vi "均衡参数输入.vi"(1 "均衡参数":T2 {"充电结束电压(100%)" min=0 max=5 format="%#.4f"; "充电结束电压(99%)" min=0 max=5 format="%#.4f"; "充电结束电压(98%)" min=0 max=5 format="%#.4f"; "充电结束电压(97%)" min=0 max=5 format="%#.4f"; "充电结束电压(96%)" min=0 max=5 format="%#.4f"; "充电结束电压(95%)" min=0 max=5 format="%#.4f"; "均衡计算-电压极差阀值" min=0 max=5 format="%#.4f"; "均衡停止-最低电压阀值" min=0 max=5 format="%#.4f"; "均衡计算-最低电压阀值" min=0 max=5 format="%#.4f"; "均衡计算-电压低阀值2级" min=0 max=5 format="%#.4f"; "充电结束电压(94%)" min=0 max=5 format="%#.4f"; "充电结束电压(93%)" min=0 max=5 format="%#.4f"; "均衡计算-电压低阀值1级" min=0 max=5 format="%#.4f"; "均衡计算-电压高阀值1级" min=0 max=5 format="%#.4f"; "均衡计算-电压高阀值2级" min=0 max=5 format="%#.4f"; "充电结束电压(92%)" min=0 max=5 format="%#.4f"; "充电结束电压(91%)" min=0 max=5 format="%#.4f"; "充电结束电压(90%)" min=0 max=5 format="%#.4f"}) -> (0 "均衡参数 2":T1 {"充电结束电压(100%)" min=0 max=5 format="%#.4f"; "充电结束电压(99%)" min=0 max=5 format="%#.4f"; "充电结束电压(98%)" min=0 max=5 format="%#.4f"; "充电结束电压(97%)" min=0 max=5 format="%#.4f"; "充电结束电压(96%)" min=0 max=5 format="%#.4f"; "充电结束电压(95%)" min=0 max=5 format="%#.4f"; "均衡计算-电压极差阀值" min=0 max=5 format="%#.4f"; "均衡停止-最低电压阀值" min=0 max=5 format="%#.4f"; "均衡计算-最低电压阀值" min=0 max=5 format="%#.4f"; "均衡计算-电压低阀值2级" min=0 max=5 format="%#.4f"; "充电结束电压(94%)" min=0 max=5 format="%#.4f"; "充电结束电压(93%)" min=0 max=5 format="%#.4f"; "均衡计算-电压低阀值1级" min=0 max=5 format="%#.4f"; "均衡计算-电压高阀值1级" min=0 max=5 format="%#.4f"; "均衡计算-电压高阀值2级" min=0 max=5 format="%#.4f"; "充电结束电压(92%)" min=0 max=5 format="%#.4f"; "充电结束电压(91%)" min=0 max=5 format="%#.4f"; "充电结束电压(90%)" min=0 max=5 format="%#.4f"})   [LabVIEW 2013]
panel:
  in  "全部输入..":bool
  in  "停止":bool
  in  "确定":bool
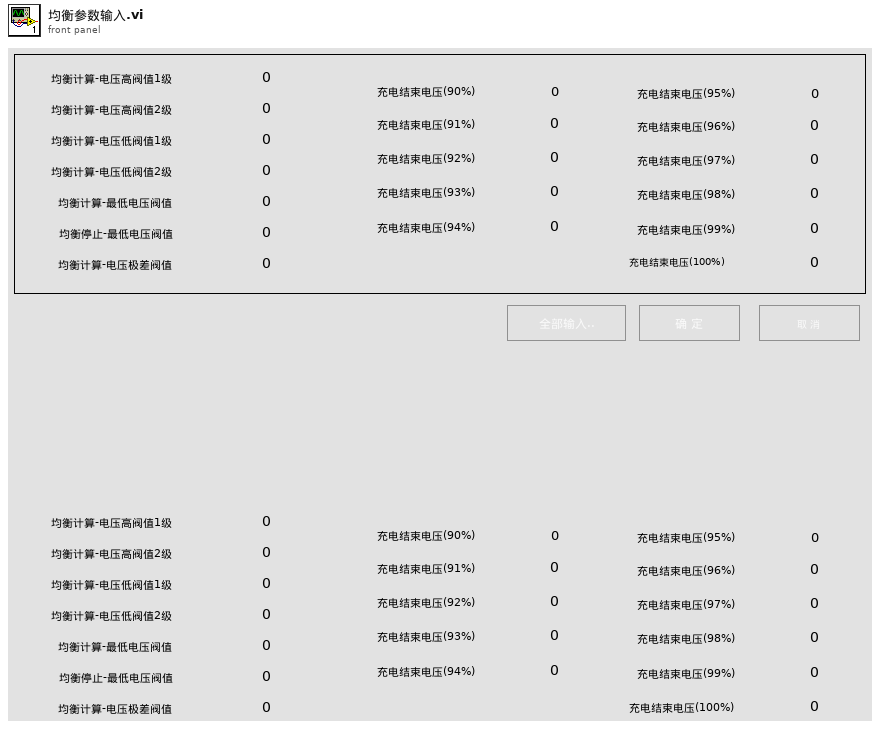
[diagram p1: front panel]
types:
  T1 = cluster{"充电结束电压(90%)":sgl, "充电结束电压(91%)":sgl, "充电结束电压(92%)":sgl, "充电结束电压(93%)":sgl, "充电结束电压(94%)":sgl, "均衡计算-电压高阀值1级":sgl, "均衡计算-电压高阀值2级":sgl, "均衡计算-电压低阀值1级":sgl, "均衡计算-电压低阀值2级":sgl, "均衡计算-最低电压阀值":sgl, "均衡停止-最低电压阀值":sgl, "均衡计算-电压极差阀值":sgl, "充电结束电压(95%)":sgl, "充电结束电压(96%)":sgl, "充电结束电压(97%)":sgl, "充电结束电压(98%)":sgl, "充电结束电压(99%)":sgl, "充电结束电压(100%)":sgl}
  T2 = cluster{"均衡计算-电压高阀值1级":sgl, "均衡计算-电压高阀值2级":sgl, "均衡计算-电压低阀值1级":sgl, "均衡计算-电压低阀值2级":sgl, "均衡计算-最低电压阀值":sgl, "均衡停止-最低电压阀值":sgl, "均衡计算-电压极差阀值":sgl, "充电结束电压(90%)":sgl, "充电结束电压(91%)":sgl, "充电结束电压(92%)":sgl, "充电结束电压(93%)":sgl, "充电结束电压(94%)":sgl, "充电结束电压(95%)":sgl, "充电结束电压(96%)":sgl, "充电结束电压(97%)":sgl, "充电结束电压(98%)":sgl, "充电结束电压(99%)":sgl, "充电结束电压(100%)":sgl}
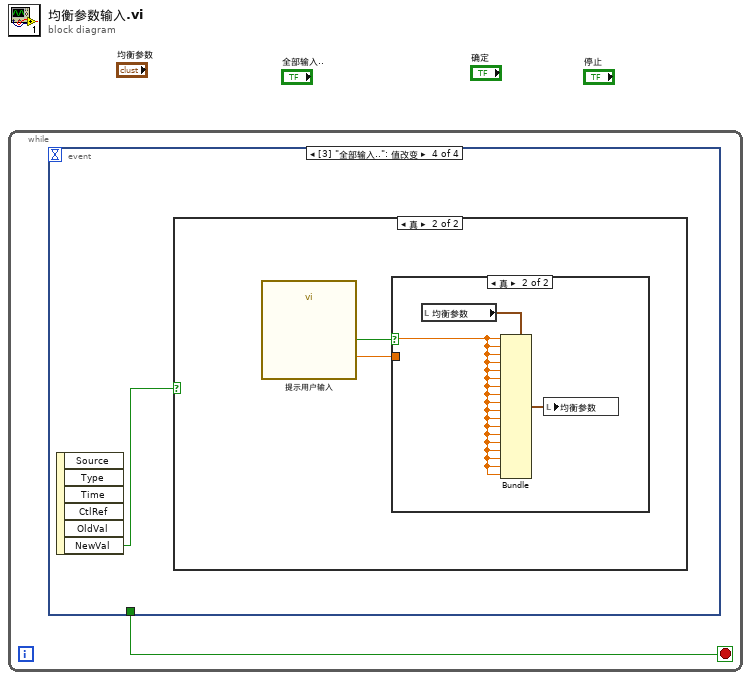
[diagram p0: block diagram]
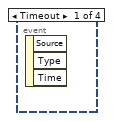
[diagram p2: hidden frame]
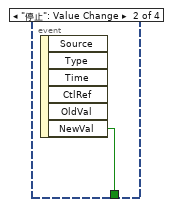
[diagram p3: hidden frame]
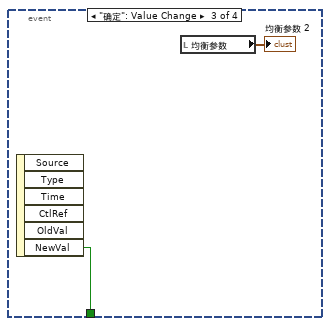
[diagram p4: hidden frame]
diagram:
  n1 = while {
    stop <- w1 stop-if-true
    n2 = event shown="[3] \"全部输入..\": 值改变" {
      selector: _ -> [_ _ _ _]
      dyn-events: _ -> [_ _ _ _]
      timeout: _ -> [_ _ _ _]
      tunnel: [_ w2 w4 _] -> w1
      event Timeout {
        n3 = event-data() -> ()  [unwired: 1 in, 3 out]
      }
      event "停止": Value Change {
        n4 = event-data() -> ("NewVal"=w2:bool)  [unwired: 1 in, 5 out]
      }
      event "确定": Value Change {
        n5 = event-data() -> ("NewVal"=w4:bool)  [unwired: 1 in, 5 out]
        n6 = local read "均衡参数"() -> (→"均衡参数 2":T2)
      }
      event "全部输入..": Value Change {
        n7 = event-data() -> ("NewVal"=w5:bool)  [unwired: 1 in, 5 out]
        n8 = case shown="真" w5 {
          frame False {
          }
          frame True {
            n9 = call "提示用户输入"() -> ("输入数值"=w6:dbl, "确定"=w7:bool)  [unwired: 17 in, 1 out]
            n10 = case shown="真" w7 {
              tunnel: w6 -> [_ w8]
              frame False {
              }
              frame True {
                n11 = local read "均衡参数"() -> (w10:T2)
                n12 = Bundle(cluster=w10, "均衡计算-电压高阀值1级"=w8, "均衡计算-电压高阀值2级"=w8, "均衡计算-电压低阀值1级"=w8, "均衡计算-电压低阀值2级"=w8, "均衡计算-最低电压阀值"=w8, "均衡停止-最低电压阀值"=w8, "均衡计算-电压极差阀值"=w8, "充电结束电压(90%)"=w8, "充电结束电压(91%)"=w8, "充电结束电压(92%)"=w8, "充电结束电压(93%)"=w8, "充电结束电压(94%)"=w8, "充电结束电压(95%)"=w8, "充电结束电压(96%)"=w8, "充电结束电压(97%)"=w8, "充电结束电压(98%)"=w8, "充电结束电压(99%)"=w8, "充电结束电压(100%)"=w8) -> (w9:T2)
                n13 = local write "均衡参数"(w9) -> ()
              }
            }
          }
        }
      }
    }
  }
